vi "Autocycle.vi"(7 "Message Queue":refnum<queue>, 8 "error in":errorcluster, 10 "Auto Para":T1={"Agitator Delays"=[], "TF Delays"=[], "Insertion Delays"=[], "Cutting Delays"=[], "PF Delays"=[], "Measur. Delays"=[1000.0], "Reject Delays"=[1000], "BF Delays"=[1000]}, 11 "Counts in":cluster{"OutputCount":u32, "RejectCount":u32}) -> (0 "error out":errorcluster, 3 "Counts out":cluster{"OutputCount":u32, "RejectCount":u32})   [LabVIEW 2017]
uses:
  Controls/Auto Delays.ctl
  support/Message Queue/Message Cluster.ctl
  Controls/Auto Times.ctl
  Global Variables/RT GV.vi
  Global Variables/FPGA GV.vi
  <vilib>/Utility/error.llb/Error Cluster From Error Code.vi
  <vilib>/rvi/errors/niLvFpgaAdjustHostInterfaceError.vi
  support/Message Queue/Enqueue Message (Single).vi
  <vilib>/rvi/interface/nirviReadWriteControl/nirviReadWriteControl.xnode
  Controls/FPGA Ref.ctl
  NiFpgaLv.dll
  <vilib>/rvi/interface/Simulation/niFpgaSimulationCallBeginRW.vi
  support/Message Queue/Message Queue.lvlib
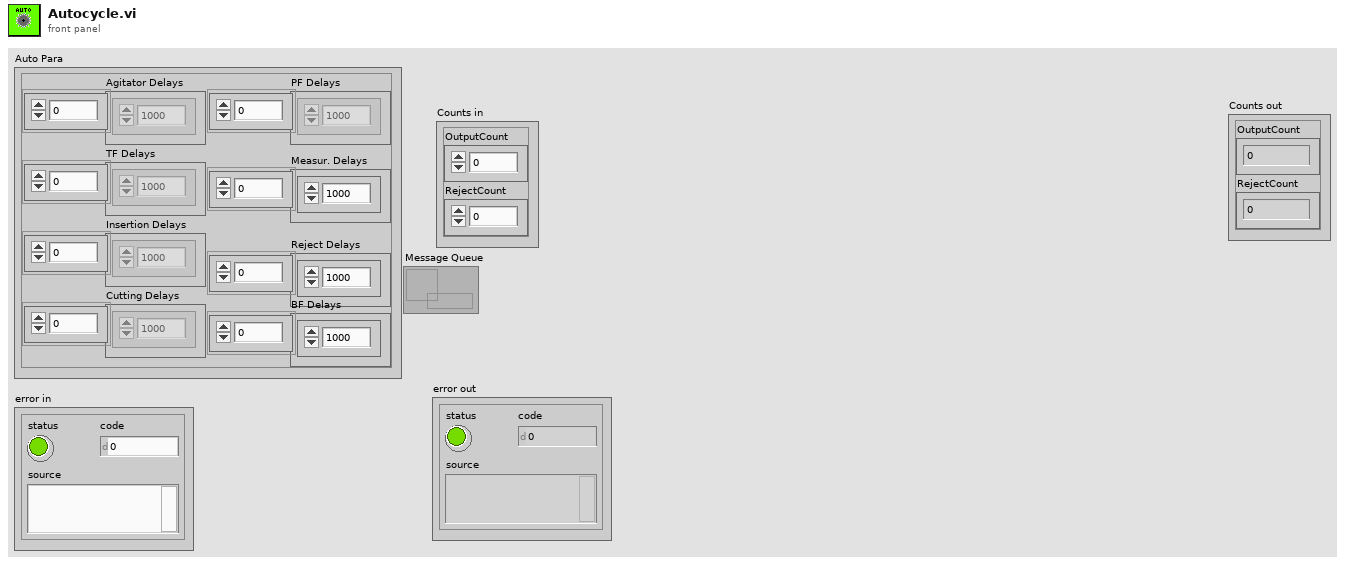
[diagram p1: front panel]
types:
  T1 = typedef "Auto Delays.ctl" = cluster{"Agitator Delays":u32[], "TF Delays":u32[], "Insertion Delays":u32[], "Cutting Delays":u32[], "PF Delays":u32[], "Measur. Delays":dbl[], "Reject Delays":u32[], "BF Delays":u32[]}
  T2 = typedef "FPGA Ref.ctl" = refnum<k20>
  T3 = cluster{"TL_Red":bool, "TL_Orange":bool, "TL_Green":bool, "TL_Buzzer":bool, "SOL_Index_Rotary_CW":bool, "SOL_Index_CNVR_Rotary_CCW":bool, "SOL_Index_CNVR_Stopper_Rear":bool, "SOL_Index_CNVR_Output _Separator _Rear":bool, "Bowl Feeder_ ON1":bool, "Pump_CNVR_Motor _ON":bool, "SOL_PC_Gating_CYL_Rear":bool, "SOL_Tube_Feed_Agitatator":bool, "SOL_Tube_Feed_Gating_CYL":bool, "SOL_Insertion _CYL":bool, "SOL_Insertion_Clamp_CYL":bool, "SOL_Cutting_CYL":bool, "SOL_Cutting_Clamp_CYL":bool, "SOL_Insertion_Air_Nozzle":bool, "SOL_Measurement_CYL":bool, "DO1.19":bool, "SOL_Rejection CYL_1":bool, "SOL_Rejection CYL_2":bool, "SOL_Rejection CYL_3":bool, "SOL_Rejection CYL_4":bool, "Bowl Feeder_ON2":bool, "SOL_BF_BlowerON":bool, "SOL_BF1_Track1":bool, "SOL_BF1_Track2":bool, "SOL_BF2_Track1":bool, "SOL_BF2_Track2":bool, "DO1.30":bool, "DO1.31":bool}
  T4 = cluster{"Indexes":i32, "seconds since 1Jan1904":timestamp}
  T5 = typedef "Auto Times.ctl" = cluster{"Index Time":u32, "TF Time":u32, "Insertion Time":u32, "Cutting Time":u32, "PF Time":u32, "Meas. Time":u32, "Reject Time":u32}
  T6 = cluster{"Reject 1":bool, "Reject 2":bool, "Reject 3":bool, "Reject 4":bool}
  T7 = cluster{"seconds since 1Jan1904":timestamp, "Auto Times":T5}
  T8 = cluster{"Reject Pallets":cluster{"Reject 1":bool, "Reject 2":bool, "Reject 3":bool, "Reject 4":bool}, "Measurements":cluster{"1":dbl, "2":dbl, "3":dbl, "4":dbl}}
  T9 = typedef "Auto Stats.ctl" = cluster{"Time":timestamp, "OEE":cluster{"AVL":dbl, "PRF":dbl, "QUA":dbl, "OEE":dbl}, "Auto Times":T5, "Counts out":cluster{"OutputCount":u32, "RejectCount":u32}, "Measurements":cluster{"1":dbl, "2":dbl, "3":dbl, "4":dbl}, "Outputs":cluster{"OutputCount":u32, "Numeric Control":u32}}
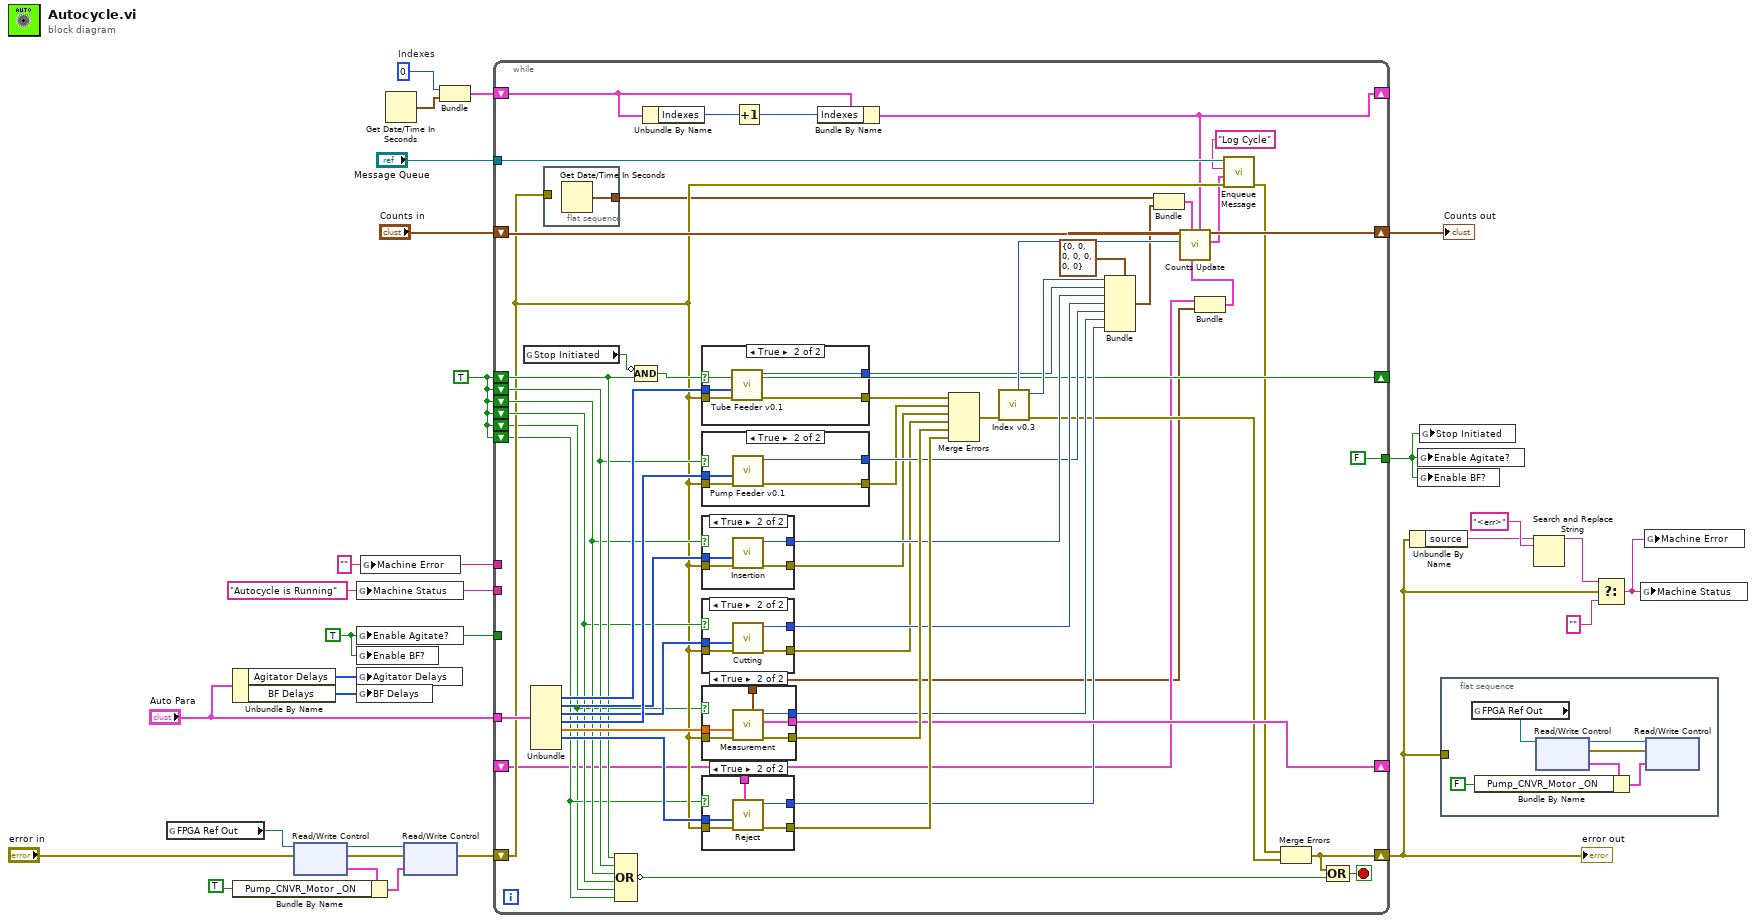
[diagram p0: block diagram]
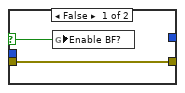
[diagram p2: hidden frame]
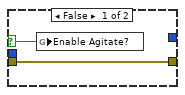
[diagram p5: hidden frame]
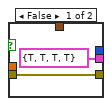
[diagram p7: hidden frame]
diagram:
  w1 = "" ("Machine Error")
  w6 = 0  # Indexes
  w12 = "Autocycle is Running" ("Machine Status")
  w23 = TRUE ("Enable Agitate?")
  w13 = TRUE
  n1 = global read "FPGA GV.vi" "FPGA Ref Out"() -> (w22:T2)
  n2 = Unbundle By Name("Auto Para") -> ("Agitator Delays"=w25:u32[], "BF Delays"=w24:u32[])
  n3 = xnode "Read/Write Control"("FPGA VI Reference In"=w22, "error in"="error in") -> ("FPGA VI Reference Out"=w17:T2, "error out"=w18:errorcluster, "DO 1"=w21:T3)
  n4 = Bundle By Name(cluster=w21, "Pump_CNVR_Motor _ON"=TRUE) -> (w20:T3)
  n5 = global write "RT GV.vi" "Machine Status"(w12) -> ()
  n6 = global write "RT GV.vi" "Enable Agitate?"(w23) -> ()
  n7 = global write "RT GV.vi" "Enable BF?"(w23) -> ()
  n8 = global write "RT GV.vi" "Agitator Delays"(w25) -> ()
  n9 = global write "RT GV.vi" "BF Delays"(w24) -> ()
  n10 = global write "RT GV.vi" "Machine Error"(w1) -> ()
  n11 = Get Date/Time In Seconds() -> (seconds since 1Jan1904=w5:timestamp)
  n12 = xnode "Read/Write Control"("FPGA VI Reference In"=w17, "error in"=w18, "DO 1"=w20) -> ("error out"=w15:errorcluster)  [unwired: 1 out]
  n13 = Bundle("Indexes"=w6, "seconds since 1Jan1904"=w5) -> (w4:T4)  [unwired: 1 in]
  n14 = while {
    tunnel: "Auto Para" -> [w78]
    shift-right: [w44] -> w10
    shift-left: w15 -> [w46]
    shift-right: [w72] -> _
    shift-left: _ -> [w38]
    shift-right: [w56] -> _
    shift-left: w13 -> [w57]
    shift-left: w13 -> [w49]
    shift-left: w13 -> [w48]
    shift-left: w13 -> [w47]
    shift-left: w13 -> [w40]
    shift-left: w13 -> [w41]
    shift-right: [w69] -> w28
    shift-left: "Counts in" -> [w68]
    tunnel: w23 -> [_]
    tunnel: "Message Queue" -> [w55]
    tunnel: [FALSE] -> w3
    tunnel: w12 -> [_]
    shift-right: [w29] -> _
    shift-left: w4 -> [w34]
    tunnel: w1 -> [_]
    stop <- w70 stop-if-true
    n15 = global read "RT GV.vi" "Stop Initiated"() -> (w58:bool)
    n16 = Unbundle(w78) -> ("TF Delays"=w81:u32[], "Insertion Delays"=w80:u32[], "Cutting Delays"=w79:u32[], "PF Delays"=w82:u32[], "Measur. Delays"=w76:dbl[], "Reject Delays"=w74:u32[])  [unwired: 2 out]
    n17 = flat-sequence {
      tunnel: w46 -> [_]
      tunnel: [w83] -> w32
      frame #0 {
        n18 = Get Date/Time In Seconds() -> (seconds since 1Jan1904=w83:timestamp)
      }
    }
    n19 = Compound Arithmetic op=OR(w57, w49, w48, w47, w40, w41) -> (invert w71:bool)
    n20 = Compound Arithmetic op=AND(invert w58, w57) -> (w56:bool)
    n21 = Unbundle By Name(w34) -> ("Indexes"=w35:i32)
    n22 = case shown="True" w56 {
      selector: w56 -> [w100 _]
      tunnel: w46 -> [w101 w105]
      tunnel: [w101 w104] -> w77
      tunnel: w81 -> [_ w103]
      tunnel: [_ w102] -> w65
      frame False {
        n23 = global write "RT GV.vi" "Enable Agitate?"(w100) -> ()
      }
      frame True {
        n24 = call "Tube Feeder v0.1.vi"("error in (no error)"=w105, "TF Para"=w103) -> ("error out"=w104:errorcluster, "TF Time"=w102:u32)  [unwired: 8 in]
      }
    }
    n25 = case shown="True" w49 {
      selector: w49 -> [w84 _]
      tunnel: w46 -> [w85 w89]
      tunnel: [w85 w88] -> w51
      tunnel: w82 -> [_ w87]
      tunnel: [_ w86] -> w62
      frame False {
        n26 = global write "RT GV.vi" "Enable BF?"(w84) -> ()
      }
      frame True {
        n27 = call "Pump Feeder v0.1.vi"("error in (no error)"=w89, "TF Delays"=w87) -> ("error out"=w88:errorcluster, "PF Time"=w86:u32)  [unwired: 8 in]
      }
    }
    n28 = case shown="True" w48 {
      tunnel: w46 -> [w95 w99]
      tunnel: [w95 w98] -> w52
      tunnel: w80 -> [_ w97]
      tunnel: [_ w96] -> w64
      frame False {
      }
      frame True {
        n29 = call "Insertion.vi"("error in (no error)"=w99, "Insertion Delays"=w97) -> ("error out"=w98:errorcluster, "Insertion Time"=w96:u32)  [unwired: 7 in, 1 out]
      }
    }
    n30 = case shown="True" w47 {
      tunnel: w46 -> [w90 w94]
      tunnel: [w90 w93] -> w53
      tunnel: w79 -> [_ w92]
      tunnel: [_ w91] -> w63
      frame False {
      }
      frame True {
        n31 = call "Cutting.vi"("error in (no error)"=w94, "Cutting Delays"=w92) -> ("error out"=w93:errorcluster, "Cutting Time"=w91:u32)  [unwired: 8 in]
      }
    }
    n32 = case shown="True" w40 {
      tunnel: w46 -> [w113 w119]
      tunnel: [w113 w118] -> w75
      tunnel: w76 -> [_ w117]
      tunnel: [_ w116] -> w61
      tunnel: [_ w115] -> w37
      tunnel: [T6 {"Reject 1"=TRUE, "Reject 2"=TRUE, "Reject 3"=TRUE, "Reject 4"=TRUE} ("Reject Pallets") w114] -> w72
      frame False {
      }
      frame True {
        n33 = call "Measurement.vi"("error in (no error)"=w119, "TF Delays"=w117) -> ("error out"=w118:errorcluster, "Reject Pallets"=w114:T6, "PF Time"=w116:u32, "Measurements"=w115:cluster{"1":dbl, "2":dbl, "3":dbl, "4":dbl})  [unwired: 6 in]
      }
    }
    n34 = case shown="True" w41 {
      tunnel: w46 -> [w106 w111]
      tunnel: [w106 w110] -> w73
      tunnel: w74 -> [_ w109]
      tunnel: [_ w108] -> w60
      tunnel: w38 -> [_ w107]
      frame False {
      }
      frame True {
        n35 = call "Reject.vi"("Reject Pallets"=w107, "error in (no error)"=w111, "TF Delays"=w109) -> ("error out"=w110:errorcluster, "PF Time"=w108:u32)  [unwired: 7 in]
      }
    }
    n36 = Increment(x=w35) -> (x+1=w33:i32)
    n37 = Bundle By Name(cluster=w34, "Indexes"=w33) -> (w29:T4)
    n38 = Merge Errors(w77, w51, w52, w53, w75, w73) -> (w45:errorcluster)
    n39 = call "Index v0.3.vi"("error in (no error)"=w45) -> ("error out"=w43:errorcluster, "Index Time"=w66:u32, "OutputCount"=w67:u32)  [unwired: 7 in, 1 out]
    n40 = Bundle(cluster=T5 {"Index Time"=0, "TF Time"=0, "Insertion Time"=0, "Cutting Time"=0, "PF Time"=0, "Meas. Time"=0, "Reject Time"=0} ("Auto Times"), "Index Time"=w66, "TF Time"=w65, "Insertion Time"=w64, "Cutting Time"=w63, "PF Time"=w62, "Meas. Time"=w61, "Reject Time"=w60) -> (w31:T5)
    n41 = Bundle("seconds since 1Jan1904"=w32, "Auto Times"=w31) -> (w30:T7)  [unwired: 1 in]
    n42 = Bundle("Reject Pallets"=w38, "Measurements"=w37) -> (w36:T8)  [unwired: 1 in]
    n43 = call "Counts Update.vi"("Perf"=w29, "output cluster"=w36, "Cluster"=w30, "OutputCount"=w67, "Counts in"=w68) -> ("Auto Stats"=w39:T9, "Counts out"=w69:cluster{"OutputCount":u32, "RejectCount":u32})  [unwired: 4 in, 1 out]
    n44 = call-poly "Enqueue Message.vi"("error in (no error)"=w46, "Message Data"=w39, "Message"="Log Cycle", "Message Queue"=w55) -> ("error out"=w42:errorcluster)  [unwired: 6 in, 1 out]
    n45 = Merge Errors(w42, w43) -> (w44:errorcluster)
    n46 = Compound Arithmetic op=OR(w44, w71) -> (w70:bool)
  }
  "error out" <- w10
  "Counts out" <- w28
  n47 = Unbundle By Name(w10) -> ("source"=w8:string)
  n48 = global write "RT GV.vi" "Enable Agitate?"(w3) -> ()
  n49 = global write "RT GV.vi" "Enable BF?"(w3) -> ()
  n50 = global write "RT GV.vi" "Stop Initiated"(w3) -> ()
  n51 = flat-sequence {
    tunnel: w10 -> [_]
    frame #0 {
      n52 = global read "FPGA GV.vi" "FPGA Ref Out"() -> (w120:T2)
      n53 = xnode "Read/Write Control"("FPGA VI Reference In"=w120) -> ("FPGA VI Reference Out"=w125:T2, "error out"=w124:errorcluster, "DO 1"=w122:T3)  [unwired: 1 in]
      n54 = Bundle By Name(cluster=w122, "Pump_CNVR_Motor _ON"=FALSE) -> (w123:T3)
      n55 = xnode "Read/Write Control"("FPGA VI Reference In"=w125, "error in"=w124, "DO 1"=w123) -> ()  [unwired: 2 out]
    }
  }
  n56 = Search and Replace String(input string=w8, search string="<err>") -> (result string=w7:string)  [unwired: 6 in, 3 out]
  n57 = Select(t=w7, s=w10, f="" ("Machine Status")) -> (s? t:f=w2:string)
  n58 = global write "RT GV.vi" "Machine Status"(w2) -> ()
  n59 = global write "RT GV.vi" "Machine Error"(w2) -> ()
